vi "FormatDataFile.vi"(11 "Dynamic data":T1) -> (3 "appended array":string[][](array[string]))   [LabVIEW 2016]
uses:
  Dynamic_data.ctl
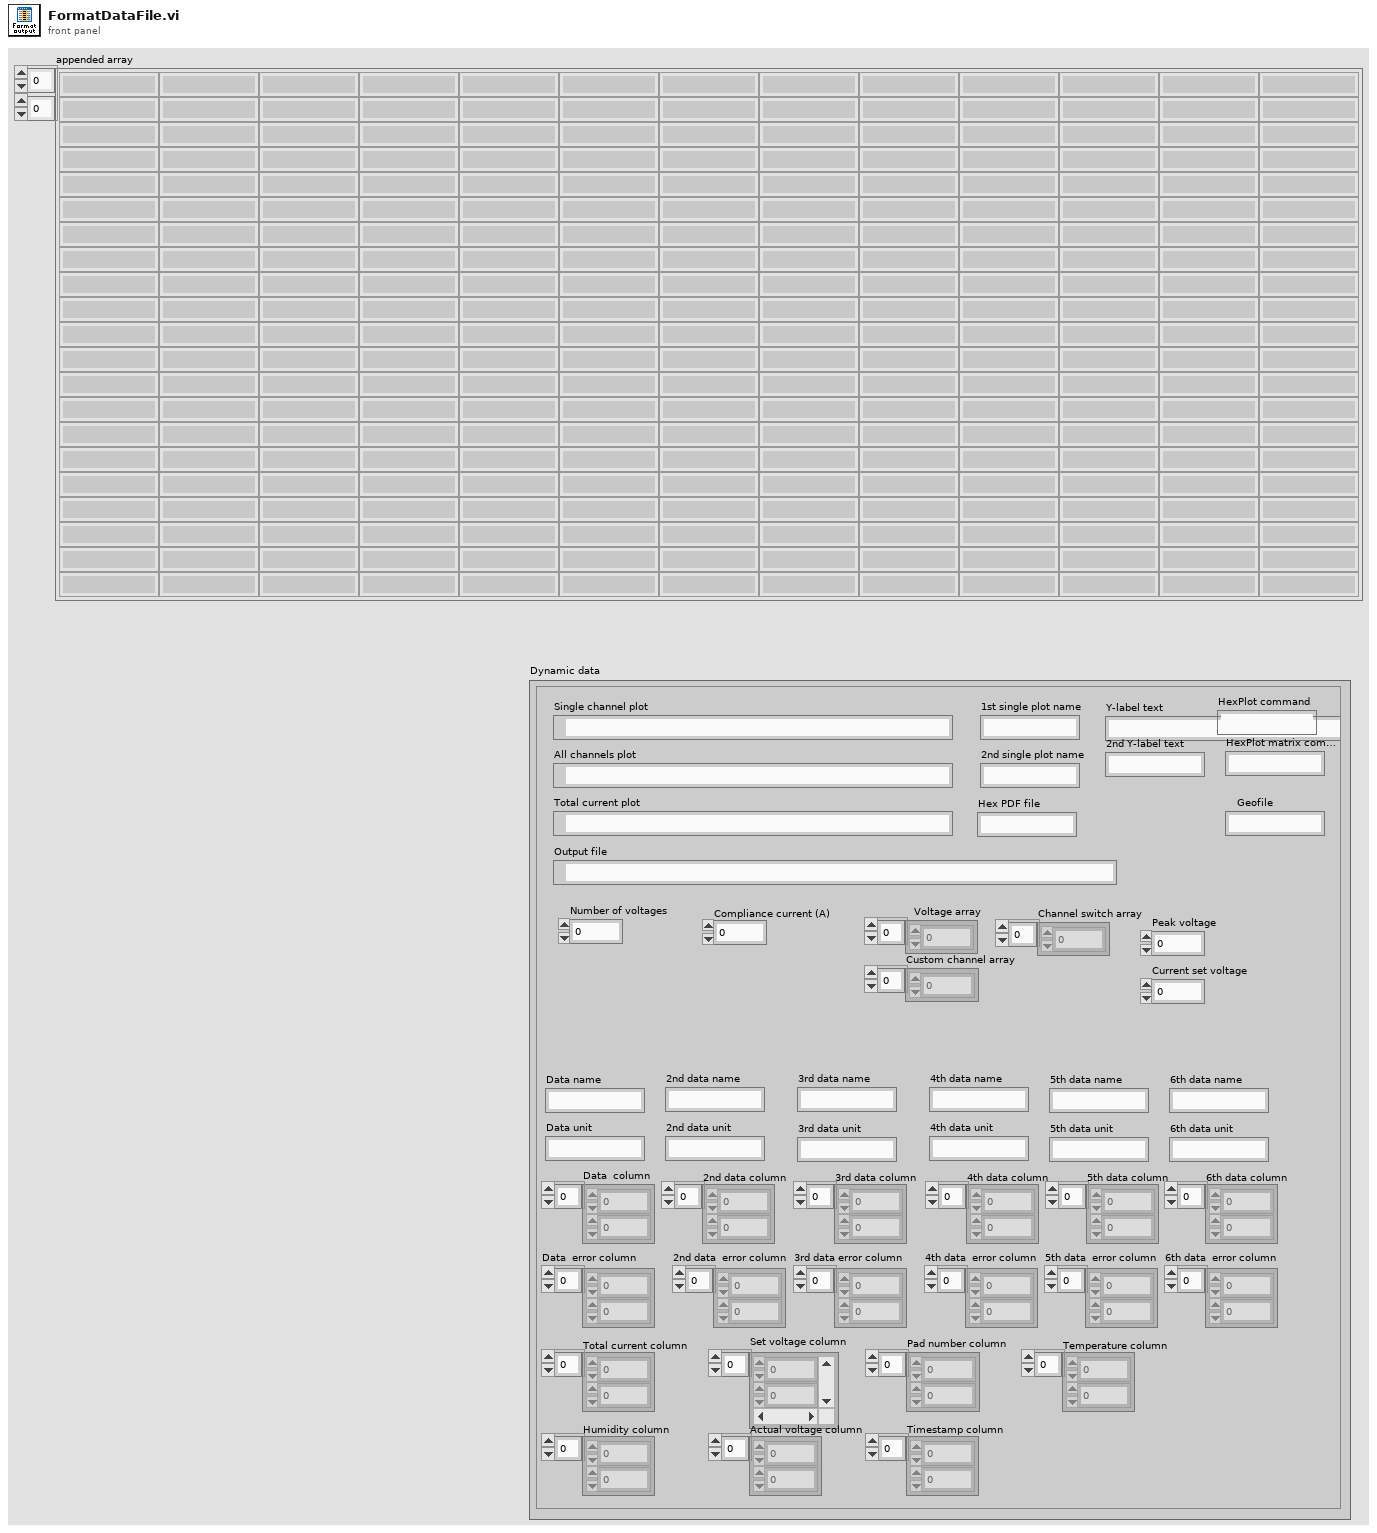
[diagram p1: front panel]
types:
  T1 = typedef "Dynamic_data.ctl" = cluster{"Output file":path, "Y-label text":string, "Current set voltage":dbl, "Set voltage column":dbl[], "Pad number column":dbl[], "Data  column":dbl[], "Number of voltages":i32, "Compliance current (A)":dbl, "Geofile":string, "Peak voltage":dbl, "Hex PDF file":string, "Voltage array":dbl[], "Total current column":dbl[], "Timestamp column":dbl[], "Data name":string, "Data unit":string, "2nd data column":dbl[], "2nd data name":string, "2nd data unit":string, "3rd data column":dbl[], "4th data column":dbl[], "3rd data name":string, "3rd data unit":string, "4th data name":string, "4th data unit":string, "Actual voltage column":dbl[], "2nd Y-label text":string, "Single channel plot":path, "Temperature column":dbl[], "Humidity column":dbl[], "Channel switch array":i32[], "1st single plot name":string, "2nd single plot name":string, "All channels plot":path, "HexPlot command":string, "Custom channel array":i32[], "Data  error column":dbl[], "2nd data  error column":dbl[], "3rd data error column":dbl[], "4th data  error column":dbl[], "Total current plot":path, "5th data column":dbl[], "5th data  error column":dbl[], "6th data column":dbl[], "6th data  error column":dbl[], "5th data name":string, "5th data unit":string, "6th data name":string, "6th data unit":string, "HexPlot matrix command":string}
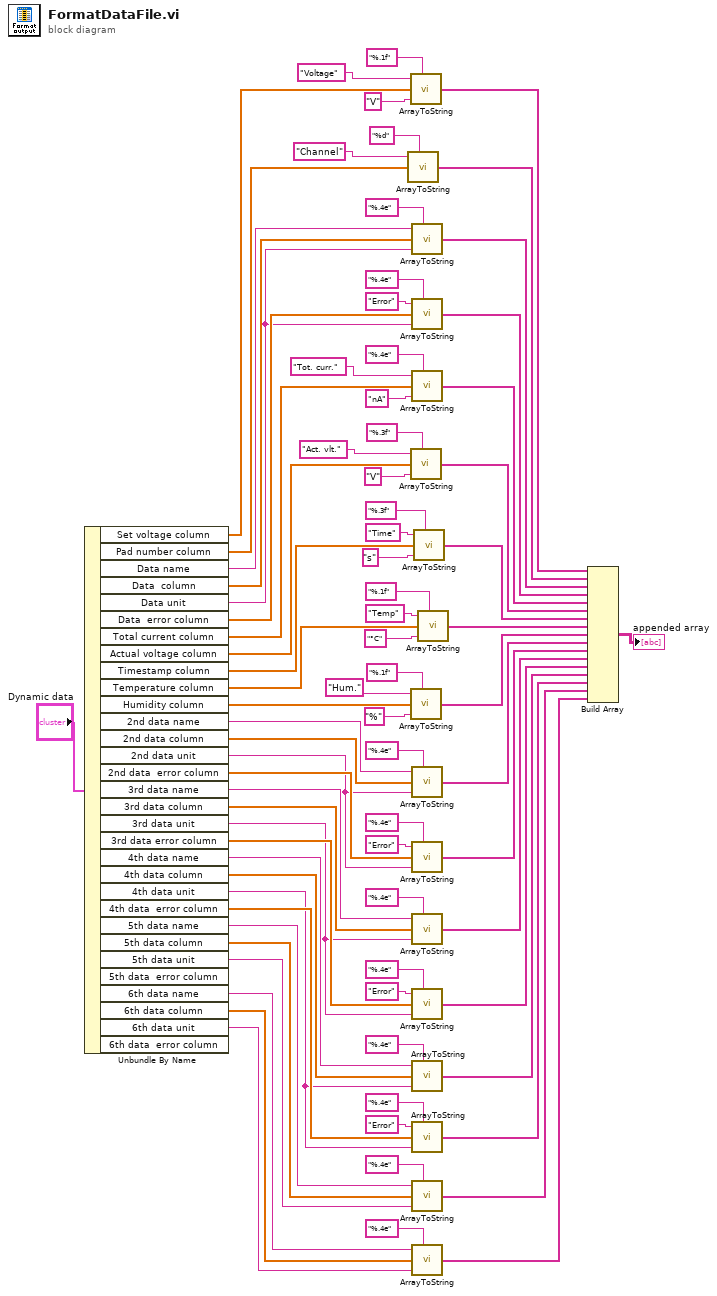
[diagram p0: block diagram]
diagram:
  n1 = Unbundle By Name("Dynamic data") -> ("Set voltage column"=w70:dbl[], "Pad number column"=w69:dbl[], "Data name"=w61:string, "Data  column"=w46:dbl[], "Data unit"=w28:string, "Data  error column"=w29:dbl[], "Total current column"=w68:dbl[], "Actual voltage column"=w42:dbl[], "Timestamp column"=w63:dbl[], "Temperature column"=w37:dbl[], "Humidity column"=w33:dbl[], "2nd data name"=w57:string, "2nd data column"=w53:dbl[], "2nd data unit"=w18:string, "2nd data  error column"=w19:dbl[], "3rd data name"=w52:string, "3rd data column"=w51:dbl[], "3rd data unit"=w16:string, "3rd data error column"=w17:dbl[], "4th data name"=w50:string, "4th data column"=w49:dbl[], "4th data unit"=w14:string, "4th data  error column"=w15:dbl[], "5th data name"=w8:string, "5th data column"=w6:dbl[], "5th data unit"=w7:string, "6th data name"=w5:string, "6th data column"=w4:dbl[], "6th data unit"=w3:string)  [unwired: 2 out]
  n2 = call "ArrayToString.vi"("Header"="Channel", "Format"="%d", "Input 1D array"=w69) -> ("Output 1D array"=w76:string[])  [unwired: 6 in]
  n3 = call "ArrayToString.vi"("Header"="Voltage", "Format"="%.1f", "Input 1D array"=w70, "Unit"="V") -> ("Output 1D array"=w77:string[])  [unwired: 5 in]
  n4 = call "ArrayToString.vi"("Header"="Act. vlt.", "Format"="%.3f", "Input 1D array"=w42, "Unit"="V") -> ("Output 1D array"=w41:string[])  [unwired: 5 in]
  n5 = call "ArrayToString.vi"("Header"="Hum.", "Format"="%.1f", "Input 1D array"=w33, "Unit"="%") -> ("Output 1D array"=w32:string[])  [unwired: 5 in]
  n6 = call "ArrayToString.vi"("Header"=w61, "Format"="%.4e", "Input 1D array"=w46, "Unit"=w28) -> ("Output 1D array"=w78:string[])  [unwired: 5 in]
  n7 = call "ArrayToString.vi"("Header"="Error", "Format"="%.4e", "Input 1D array"=w29, "Unit"=w28) -> ("Output 1D array"=w26:string[])  [unwired: 5 in]
  n8 = call "ArrayToString.vi"("Header"="Tot. curr.", "Format"="%.4e", "Input 1D array"=w68, "Unit"="nA") -> ("Output 1D array"=w71:string[])  [unwired: 5 in]
  n9 = call "ArrayToString.vi"("Header"=w57, "Format"="%.4e", "Input 1D array"=w53, "Unit"=w18) -> ("Output 1D array"=w56:string[])  [unwired: 5 in]
  n10 = call "ArrayToString.vi"("Header"="Error", "Format"="%.4e", "Input 1D array"=w19, "Unit"=w18) -> ("Output 1D array"=w13:string[])  [unwired: 5 in]
  n11 = call "ArrayToString.vi"("Header"=w52, "Format"="%.4e", "Input 1D array"=w51, "Unit"=w16) -> ("Output 1D array"=w48:string[])  [unwired: 5 in]
  n12 = call "ArrayToString.vi"("Header"="Error", "Format"="%.4e", "Input 1D array"=w17, "Unit"=w16) -> ("Output 1D array"=w12:string[])  [unwired: 5 in]
  n13 = call "ArrayToString.vi"("Header"=w50, "Format"="%.4e", "Input 1D array"=w49, "Unit"=w14) -> ("Output 1D array"=w47:string[])  [unwired: 5 in]
  n14 = call "ArrayToString.vi"("Header"="Error", "Format"="%.4e", "Input 1D array"=w15, "Unit"=w14) -> ("Output 1D array"=w11:string[])  [unwired: 5 in]
  n15 = call "ArrayToString.vi"("Header"=w8, "Format"="%.4e", "Input 1D array"=w6, "Unit"=w7) -> ("Output 1D array"=w2:string[])  [unwired: 5 in]
  n16 = call "ArrayToString.vi"("Header"=w5, "Format"="%.4e", "Input 1D array"=w4, "Unit"=w3) -> ("Output 1D array"=w1:string[])  [unwired: 5 in]
  n17 = call "ArrayToString.vi"("Header"="Time", "Format"="%.3f", "Input 1D array"=w63, "Unit"="s") -> ("Output 1D array"=w65:string[])  [unwired: 5 in]
  n18 = call "ArrayToString.vi"("Header"="Temp", "Format"="%.1f", "Input 1D array"=w37, "Unit"="°C") -> ("Output 1D array"=w31:string[])  [unwired: 5 in]
  n19 = Build Array(w77, w76, w78, w26, w71, w41, w65, w31, w32, w56, w13, w48, w12, w47, w11, w2, w1) -> (→"appended array":string[][])
